vi "Parameter Set Write Array.vi"(8 "error in":errorcluster, 10 "Control Mode STS":i32[](array[numeric]), 11 "Cycler in":refnum<class "Cycler.lvclass">) -> (0 "error out":errorcluster, 3 "Cycler out":refnum<class "Cycler.lvclass">)   [LabVIEW 2023, in "Cycler.lvclass"]
uses:
  Cycler.lvclass
  Low Level Capabilities/Parameter Set/Parameter Set.lvclass
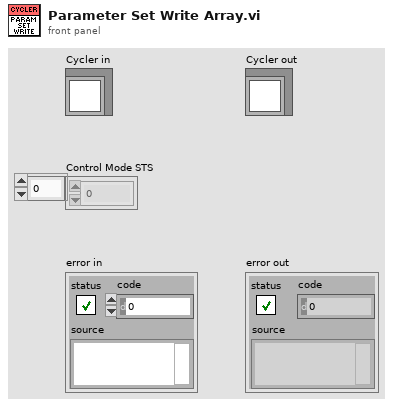
[diagram p1: front panel]
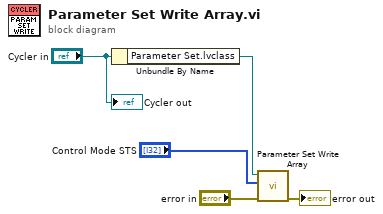
[diagram p0: block diagram]
diagram:
  n1 = Unbundle By Name("Cycler in") -> ("Parameter Set.lvclass"=w4:refnum<class "Parameter Set.lvclass">)
  n2 = call-dynamic "Parameter Set Write Array.vi"("error in"="error in", "Control Mode STS"="Control Mode STS", "Parameter Set in"=w4) -> ("error out"=→"error out":errorcluster)  [unwired: 7 in, 1 out]
  "Cycler out" <- "Cycler in"
